vi "Stop Acquisition.vi"(8 "error in (no error)":errorcluster, 11 "IMAQdx Actor in":refnum<class "IMAQdx Actor.lvclass">) -> (0 "error out":errorcluster, 3 "IMAQdx Actor out":refnum<class "IMAQdx Actor.lvclass">)   [LabVIEW 2014, in "IMAQdx Actor.lvlib" / "IMAQdx Actor.lvclass"]
uses:
  IMAQdx Actor.lvclass
  <vilib>/userdefined/High Color/IMAQdx.ctl
  <vilib>/vision/Image Controls.llb/IMAQ Image.ctl
  IMAQdx Actor.lvclass/IMAQdx Actor.ctl
  <vilib>/vision/driver/NI_Vision_Acquisition_Software.lvlib
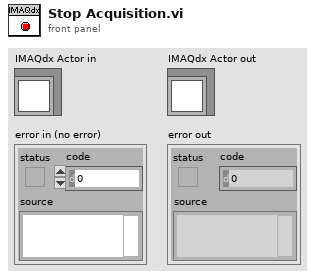
[diagram p1: front panel]
types:
  T1 = typedef "IMAQ Image.ctl" = refnum<image>
  T2 = typedef "IMAQdx.ctl" = refnum<k21>
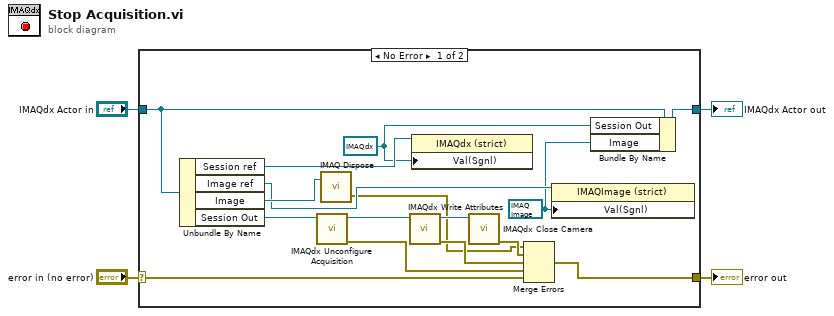
[diagram p0: block diagram]
diagram:
  n1 = case shown="No Error" "error in (no error)" {
    selector: "error in (no error)" -> [w13 w22]
    tunnel: [w12 w22] -> w3
    tunnel: [w9 w21] -> w1
    tunnel: "IMAQdx Actor in" -> [w17 w21]
    frame No Error {
      w6 = T1 refnum ("Value (Signaling)")
      w8 = T2 refnum ("Session Out")
      n2 = Unbundle By Name(w17) -> ("Session ref"=w10:refnum<vi>, "Image ref"=w7:refnum<vi>, "Image"=w11:T1, "Session Out"=w18:T2)
      n3 = call <vilib>:"IMAQdx Unconfigure Acquisition.vi"("Session In"=w18) -> ("error out"=w15:errorcluster, "Session Out"=w19:T2)  [unwired: 1 in, 8 out]
      n4 = call "IMAQ Dispose"("Image"=w11) -> ("error out"=w5:errorcluster)  [unwired: 5 in]
      n5 = call <vilib>:"IMAQdx Write Attributes.vi"("Session In"=w19) -> ("error out"=w14:errorcluster, "Session Out"=w20:T2)  [unwired: 9 in]
      n6 = property class="IMAQdx (strict)"(reference=w10, "Val(Sgnl)"=w8) -> ()  [unwired: 1 in, 2 out]
      n7 = call <vilib>:"IMAQdx Close Camera.vi"("Session In"=w20) -> ("error out"=w16:errorcluster)  [unwired: 1 in, 9 out]
      n8 = Merge Errors(w5, w16, w14, w15, w13) -> (w12:errorcluster)
      n9 = property class="IMAQImage (strict)"(reference=w7, "Val(Sgnl)"=w6) -> ()  [unwired: 1 in, 2 out]
      n10 = Bundle By Name(cluster=w17, "Session Out"=w8, "Image"=w6) -> (w9:refnum<class "IMAQdx Actor.lvclass">)
    }
    frame Error {
    }
  }
  "error out" <- w3
  "IMAQdx Actor out" <- w1
